vi "Remove all spaces and tabs from string.vi"(1 "String in":string) -> (0 "String out":string)   [LabVIEW 2013]
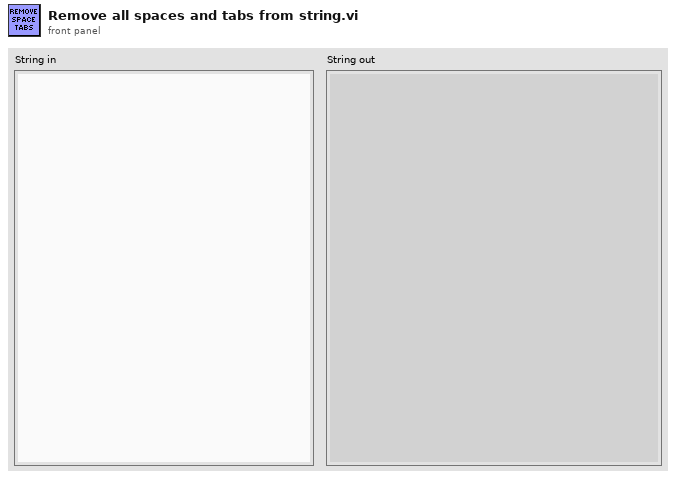
[diagram p1: front panel]
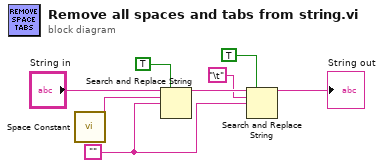
[diagram p0: block diagram]
diagram:
  w4 = ""
  n1 = call <vilib>:"Space Constant.vi"() -> ("String"=w6:string)
  n2 = Search and Replace String(replace all?=TRUE ("replace all? (F)"), input string="String in", search string=w6, replace string=w4) -> (result string=w5:string)  [unwired: 4 in, 3 out]
  n3 = Search and Replace String(replace all?=TRUE ("replace all? (F)"), input string=w5, search string="\t", replace string=w4) -> (result string=→"String out":string)  [unwired: 4 in, 3 out]
